vi "Automated Controllers Test.vi"() -> ()   [LabVIEW 2020, in "Hardware Abstraction App.lvclass"]
uses:
  Hardware Abstraction App/Hardware Abstraction App.lvclass
  Factories/Automated Controller/Automated Controller.lvclass
  Devices/AutomatedController/AutomatedController.lvclass
  Devices/PLC/PLC.lvclass
  Devices/OPC/OPC.lvclass
  Devices/cRIO/cRIO.lvclass
  Devices/ESP8266/ESP8266.lvclass
  Devices/Arduino/Arduino.lvclass
  Accessories/Wi-Fi Shield/Wi-Fi Shield.lvclass
  C:/Users/fflores/Documents/GitHub Projects/HAL-with-Interfaces/Interfaces/Arduino Shield/Arduino Shield.lvclass
  C:/Users/fflores/Documents/GitHub Projects/HAL-with-Interfaces/Devices/AutomatedController/AutomatedController.lvclass
panel:
  in  "Stop Button":bool
  in  "Dispositivo":i32(listbox)=3
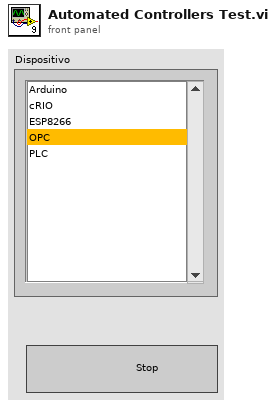
[diagram p1: front panel]
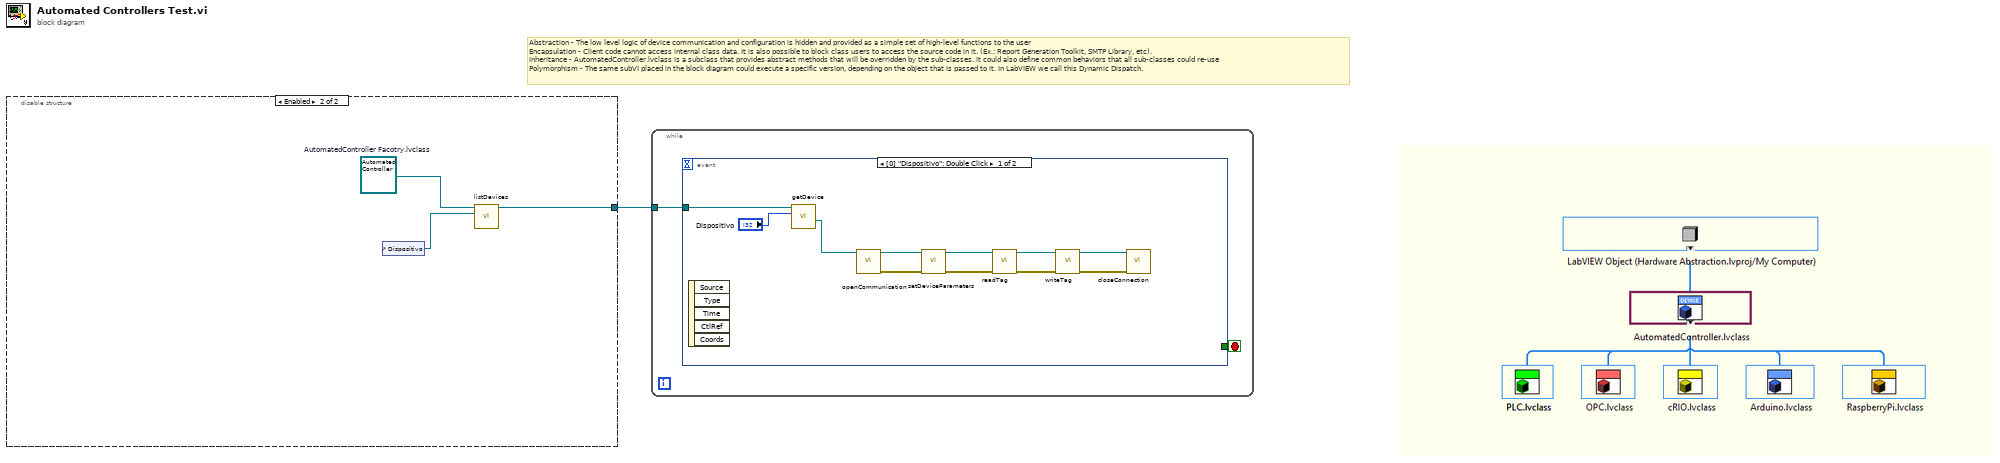
[diagram p0: block diagram]
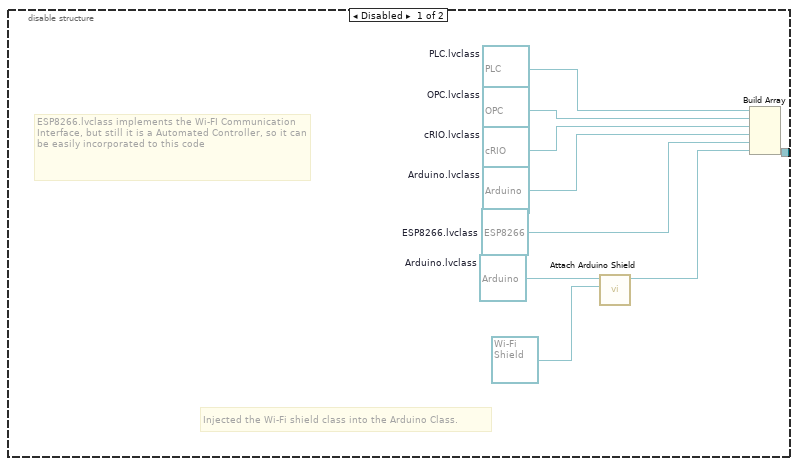
[diagram p2: hidden frame]
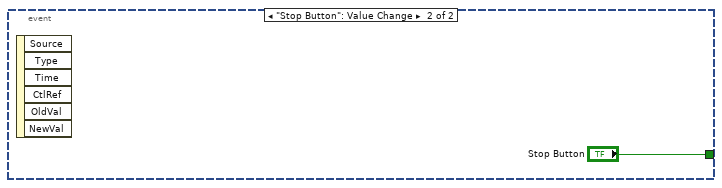
[diagram p3: hidden frame]
diagram:
  # "Abstraction - The low level logic of device communication and configuration is hidden and provided as a simple set of high-level functions to the user\nEncapsulation - Client code cannot access internal class data. It is also possible to block class users to access the source code in it. (Ex.: Report Generation Toolkit, SMTP Library, etc).\nInheritance - AutomatedController.lvclass is a subclass that provides abstract methods that will be overridden by the sub-classes. it could also define common behaviors that all sub-classes could re-use\nPolymorphism - The same subVI placed in the block diagram could execute a specific version, depending on the object that is passed to it. In LabVIEW we call this Dynamic Dispatch."
  n1 = disable-structure shown="Enabled" {
    disable-tunnel: [_ w11] -> w1
    frame Disabled {
      w4 = refnum<class "Arduino.lvclass"> refnum  # Arduino.lvclass
      w9 = refnum<class "PLC.lvclass"> refnum  # PLC.lvclass
      w8 = refnum<class "OPC.lvclass"> refnum  # OPC.lvclass
      w7 = refnum<class "cRIO.lvclass"> refnum  # cRIO.lvclass
      w6 = refnum<class "Arduino.lvclass"> refnum  # Arduino.lvclass
      w5 = refnum<class "ESP8266.lvclass"> refnum  # ESP8266.lvclass
      # "Injected the Wi-Fi shield class into the Arduino Class."
      # "ESP8266.lvclass implements the Wi-FI Communication Interface, but still it is a Automated Controller, so it can be easily incorporated to this code"
      n2 = call "Attach Arduino Shield.vi"("Arduino Shield"=refnum<class "Wi-Fi Shield.lvclass"> refnum ("Wi-Fi Shield.lvclass"), "Arduino in"=w4) -> ("Arduino out"=w3:refnum<class "Arduino.lvclass">)  [unwired: 8 in, 1 out]
      n3 = Build Array(w9, w8, w7, w6, w5, w3) -> ()  [unwired: 1 out]
    }
    frame Enabled {
      w10 = refnum<class "Automated Controller.lvclass"> refnum  # AutomatedController Facotry.lvclass
      n4 = control-ref of="Dispositivo"() -> (w12:refnum<vi>)
      n5 = call-dynamic "listDevices.vi"("Listbox Reference"=w12, "DeviceFactory in"=w10) -> ("DeviceFactory out"=w11:refnum<class "Automated Controller.lvclass">)  [unwired: 8 in, 1 out]
    }
  }
  n6 = while {
    tunnel: w1 -> [w13]
    stop <- w14 stop-if-true
    n7 = event shown="[0] \"Dispositivo\": Double Click" {
      selector: _ -> [_ _]
      dyn-events: _ -> [_ _]
      timeout: _ -> [_ _]
      tunnel: [_ "Stop Button"] -> w14
      tunnel: w13 -> [w17 _]
      event "Dispositivo": Double Click {
        n8 = event-data() -> ()  [unwired: 1 in, 5 out]
        n9 = call-dynamic "getDevice.vi"("Device Number"="Dispositivo", "DeviceFactory in"=w17) -> ("AutomatedController"=w15:refnum<class "AutomatedController.lvclass">)  [unwired: 7 in, 2 out]
        n10 = call-dynamic "openCommunication.vi"("AutomatedController in"=w15) -> ("error out"=w24:errorcluster, "AutomatedController out"=w25:refnum<class "AutomatedController.lvclass">)  [unwired: 9 in]
        n11 = call-dynamic "setDeviceParameters.vi"("error in (no error)"=w24, "AutomatedController in"=w25) -> ("error out"=w23:errorcluster, "AutomatedController out"=w18:refnum<class "AutomatedController.lvclass">)  [unwired: 8 in]
        n12 = call-dynamic "readTag.vi"("error in (no error)"=w23, "AutomatedController in"=w18) -> ("error out"=w21:errorcluster, "AutomatedController out"=w22:refnum<class "AutomatedController.lvclass">)  [unwired: 8 in]
        n13 = call-dynamic "writeTag.vi"("error in (no error)"=w21, "AutomatedController in"=w22) -> ("error out"=w19:errorcluster, "AutomatedController out"=w20:refnum<class "AutomatedController.lvclass">)  [unwired: 8 in]
        n14 = call-dynamic "closeConnection.vi"("error in (no error)"=w19, "AutomatedController in"=w20) -> ()  [unwired: 8 in, 2 out]
      }
      event "Stop Button": Value Change {
        n15 = event-data() -> ()  [unwired: 1 in, 6 out]
      }
    }
  }
